vi "LIN EX Master Stop Sch.vi"(10 "LINIndex":u8, 11 "DevHandle":i32) -> (3 "function return":i32)   [LabVIEW 2010, in "usb2lin_ex.lvlib"]
doc: "int WINAPI LIN_EX_MasterStopSch(int DevHandle,unsigned char LINIndex);"
uses:
  usb2lin_ex.lvlib
  USB2XXX.dll
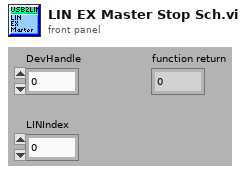
[diagram p1: front panel]
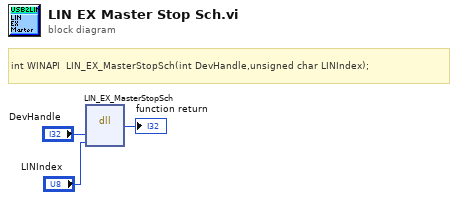
[diagram p0: block diagram]
diagram:
  # "int WINAPI  LIN_EX_MasterStopSch(int DevHandle,unsigned char LINIndex);"
  n1 = dll-call lib="E:/OtherWork/STM32/USB2XXX_Example/sdk/api/Labview/USB2XXX.*" fn="LIN_EX_MasterStopSch"("DevHandle"="DevHandle", "LINIndex"="LINIndex") -> (→"function return":i32)  [unwired: 5 in, 2 out]
